vi "SaveFinger.vi"(8 "error in (no error)":errorcluster, 11 "Finger Refnum":refnum<k24>) -> (0 "error out":errorcluster, 3 "Finger":T1)   [LabVIEW 2017, in "LeapMotion.lvlib"]
uses:
  LeapMotion.lvlib
  TypeDefs/LEAPfinger.ctl
  TypeDefs/LEAPvector.ctl
  TypeDefs/LEAPbone.ctl
  C:/Users/snordinh/Desktop/LEAP/LEAP-sign-language-test/LeapMotion/Dynamic Libraries/LeapCSharp.NET4.5.dll
  Dynamic Libraries/LeapCSharp.NET4.5.dll
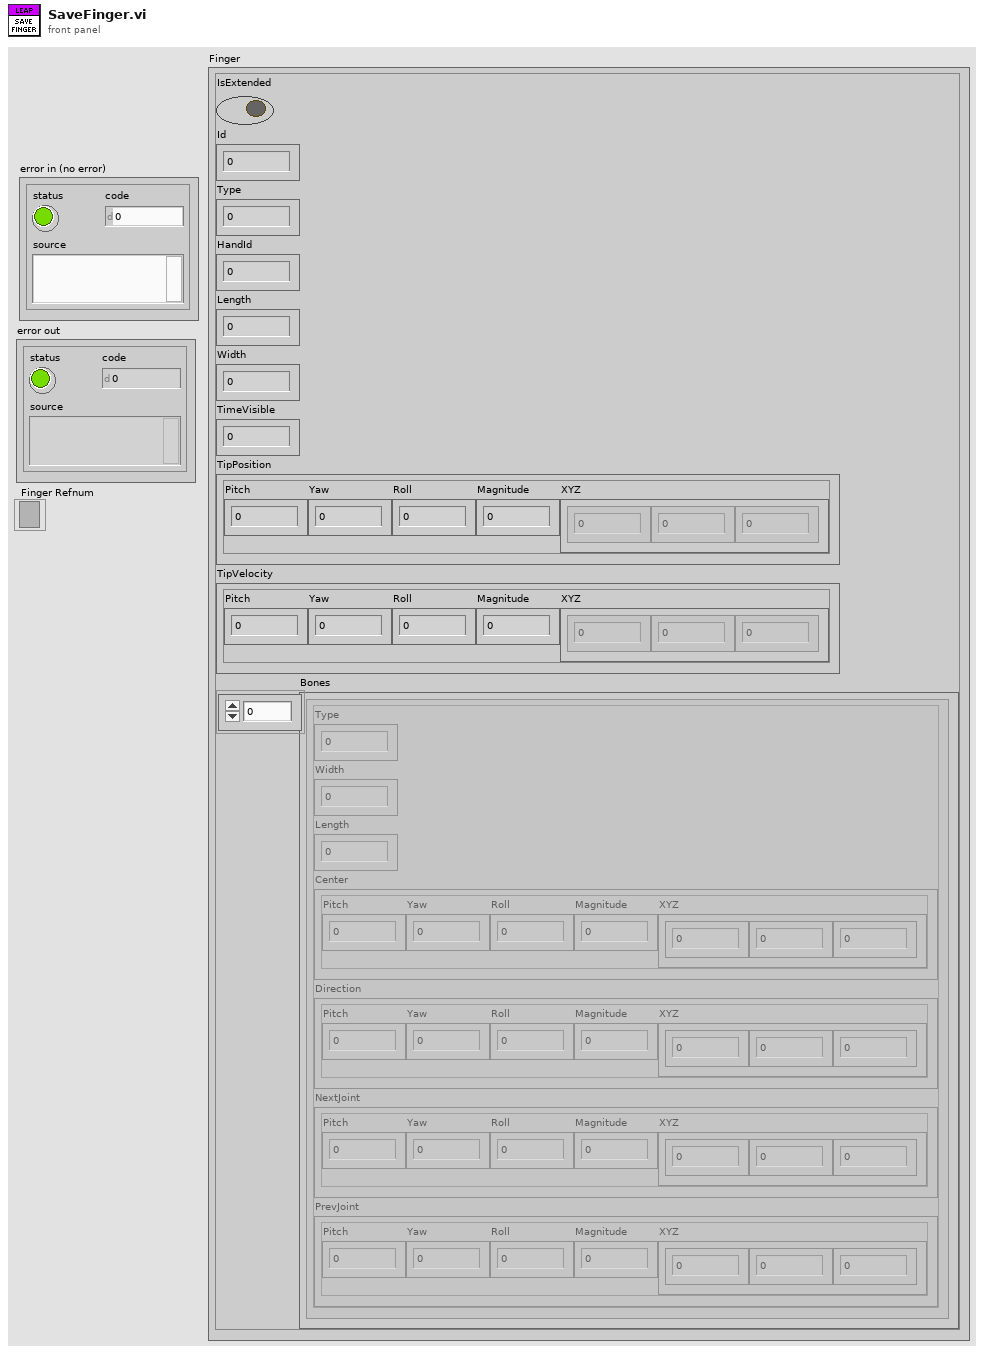
[diagram p1: front panel]
types:
  T1 = typedef "LeapMotion.lvlib/LEAPfinger.ctl" = cluster{"IsExtended":bool, "Id":i32, "Type":i32, "HandId":i32, "Length":sgl, "Width":sgl, "TimeVisible":sgl, "TipPosition":T2, "TipVelocity":T2, "Bones":T3[]}
  T2 = typedef "LeapMotion.lvlib/LEAPvector.ctl" = cluster{"Pitch":sgl, "Yaw":sgl, "Roll":sgl, "Magnitude":sgl, "XYZ":sgl[]}
  T3 = typedef "LeapMotion.lvlib/LEAPbone.ctl" = cluster{"Type":i32, "Width":sgl, "Length":sgl, "Center":T2, "Direction":T2, "NextJoint":T2, "PrevJoint":T2}
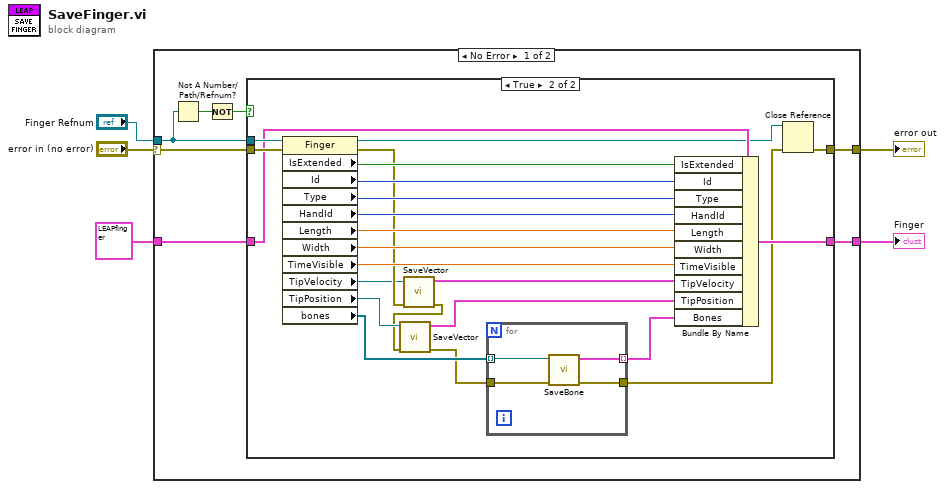
[diagram p0: block diagram]
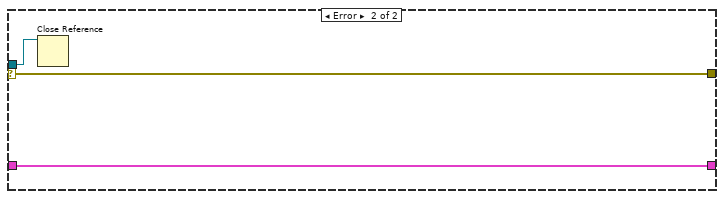
[diagram p3: hidden frame]
diagram:
  n1 = case shown="No Error" "error in (no error)" {
    selector: "error in (no error)" -> [w6 w42]
    tunnel: [w12 w42] -> w2
    tunnel: "Finger Refnum" -> [w7 w44]
    tunnel: [w11 w43] -> w1
    tunnel: T1 {"IsExtended"=FALSE, "Id"=0, "Type"=0, "HandId"=0, "Length"=0.0, "Width"=0.0, "TimeVisible"=0.0, "TipPosition"={"Pitch"=0.0, "Yaw"=0.0, "Roll"=0.0, "Magnitude"=0.0, "XYZ"=[]}, "TipVelocity"={"Pitch"=0.0, "Yaw"=0.0, "Roll"=0.0, "Magnitude"=0.0, "XYZ"=[]}, "Bones"=[]} ("Finger") -> [w10 w43]
    frame No Error {
      n2 = Not A Number/Path/Refnum?(number/path/refnum=w7) -> (NaN/Path/Refnum?=w9:bool)
      n3 = Not(x=w9) -> (.not. x?=w8:bool)
      n4 = case shown="True" w8 {
        tunnel: [w14 w24] -> w12
        tunnel: w6 -> [w14 w37]
        tunnel: w7 -> [_ w36]
        tunnel: [w13 w28] -> w11
        tunnel: w10 -> [w13 w27]
        frame False {
        }
        frame True {
          n5 = property class="Finger"(reference=w36, error in=w37) -> (reference out=w26:refnum<k24>, error out=w18:errorcluster, "IsExtended"=w35:bool, "Id"=w34:i32, "Type"=w33:i32, "HandId"=w32:i32, "Length"=w31:sgl, "Width"=w30:sgl, "TimeVisible"=w29:sgl, "TipVelocity"=w17:refnum<k24>, "TipPosition"=w22:refnum<k24>, "bones"=w23:refnum<k24>[])
          n6 = call "SaveVector.vi"("error in (no error)"=w18, "Vector Refnum"=w17) -> ("error out"=w15:errorcluster, "LEAPvector"=w16:T2)  [unwired: 8 in]
          n7 = call "SaveVector.vi"("error in (no error)"=w15, "Vector Refnum"=w22) -> ("error out"=w19:errorcluster, "LEAPvector"=w20:T2)  [unwired: 8 in]
          n8 = for {
            tunnel: w23 -> [w38] mode=indexing
            tunnel: [w39] -> w21 mode=indexing
            tunnel: w19 -> [w40]
            tunnel: [w41] -> w25
            n9 = call "SaveBone.vi"("error in (no error)"=w40, "Bone Refnum"=w38) -> ("error out"=w41:errorcluster, "Bone"=w39:T3)  [unwired: 8 in]
          }
          n10 = Bundle By Name(cluster=w27, "IsExtended"=w35, "Id"=w34, "Type"=w33, "HandId"=w32, "Length"=w31, "Width"=w30, "TimeVisible"=w29, "TipVelocity"=w16, "TipPosition"=w20, "Bones"=w21) -> (w28:T1)
          n11 = Close Reference(reference=w26, error in (no error)=w25) -> (error out=w24:errorcluster)
        }
      }
    }
    frame Error {
      n12 = Close Reference(reference=w44) -> ()  [unwired: 1 in, 1 out]
    }
  }
  "Finger" <- w1
  "error out" <- w2
